vi "UIWriteCtrlArray.vi"(8 "error in":errorcluster, 9 "Control Value":variant[](array[variant]), 10 "Control Label":string[](array[string]), 11 "UI Ref cluster in":T1) -> (0 "error out":errorcluster, 3 "UI Ref cluster out":T1)   [LabVIEW 2025, in "UI_Library.lvlib" / "UI_Library.lvclass"]
doc: "Write new value to all Controls if found"
uses:
  UI_Library.lvclass
  Controls/UI_RefCluster.ctl
  <vilib>/Utility/Data Type/Type Definitions/Data Type.ctl
  UI_Library.lvlib
  <vilib>/Utility/Data Type/NI_Data Type.lvlib
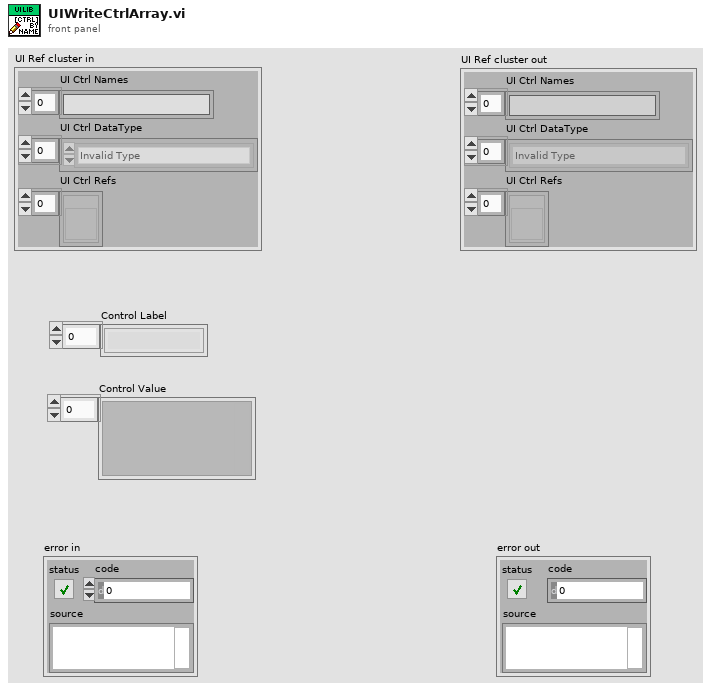
[diagram p1: front panel]
types:
  T1 = typedef "UI_Library.lvlib/UI_RefCluster.ctl" = cluster{"UI Ctrl Names":string[], "UI Ctrl DataType":T2[], "UI Ctrl Refs":refnum<vi>[]}
  T2 = typedef "NI_Data Type.lvlib/Data Type.ctl" = enum8{"Invalid Type", "Void", "I8", "I16", "I32", "I64", "U8", "U16", "U32", "U64", "Single Float", "Double Float", "Extended Float", "Single Complex", "Double Complex", "Extended Complex", "Enum U8", "Enum U16", "Enum U32", "Enum U64", "Single Float With Unit", "Double Float With Unit", "Extended Float With Unit", "Single Complex with Unit", "Double Complex with Unit", "Extended Complex with Unit", "Boolean", "String", "Path", "Picture", "Tag", "Array", "Cluster", "Variant", "LV Variant", "Waveform", "Timestamp", "Digital Waveform", "Digital Data", "ExpressData", "Refnum", "External Data", "VI", "Poly VI", "LabVIEW Class Instance", "Fixed Point", "Set Collection", "Map Collection"}
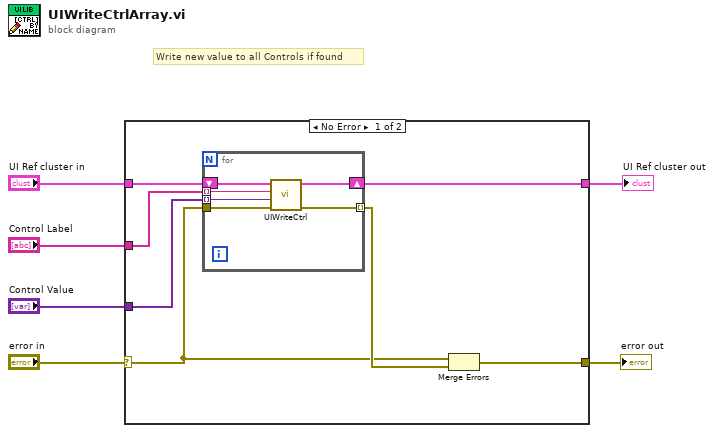
[diagram p0: block diagram]
diagram:
  # "Write new value to all Controls if found"
  n1 = case shown="No Error" "error in" {
    selector: "error in" -> [w7 w21]
    tunnel: [w8 w21] -> w6
    tunnel: "Control Value" -> [w10 _]
    tunnel: "Control Label" -> [w11 _]
    tunnel: [w12 w20] -> w2
    tunnel: "UI Ref cluster in" -> [w13 w20]
    frame No Error {
      n2 = for {
        tunnel: w11 -> [w15] mode=indexing
        tunnel: w10 -> [w14] mode=indexing
        shift-right: [w18] -> w12
        shift-left: w13 -> [w19]
        tunnel: w7 -> [w17]
        tunnel: [w16] -> w9 mode=indexing
        n3 = call "UIWriteCtrl.vi"("error in"=w17, "Control Value"=w14, "Control Label"=w15, "UI Ref cluster in"=w19) -> ("error out"=w16:errorcluster, "UI Ref cluster out"=w18:T1)  [unwired: 6 in]
      }
      n4 = Merge Errors(w7, w9) -> (w8:errorcluster)
    }
    frame Error {
    }
  }
  "error out" <- w6
  "UI Ref cluster out" <- w2
